vi "Force and Diameter Charts Notifier Debug.vi"(8 "error in (no error)":errorcluster, 9 "gui notifier":refnum<notifier>, 10 "error queue":refnum<queue>, 11 "ia test notifier":refnum<notifier>) -> (0 "error out":errorcluster)   [LabVIEW 2020]
uses:
  GUI/Main GUI Loop/Handler.ctl
  Inflation Test/Result Handling/Inflation Test Numeric Results.ctl
panel:
  out "diameter":cluster{dbl[], dbl[]}(graph)
  out "force vs setpoint":cluster{dbl[], dbl[]}[](graph)
  # "DIAMETER"
  # "FORCE VS. SETPOINT"
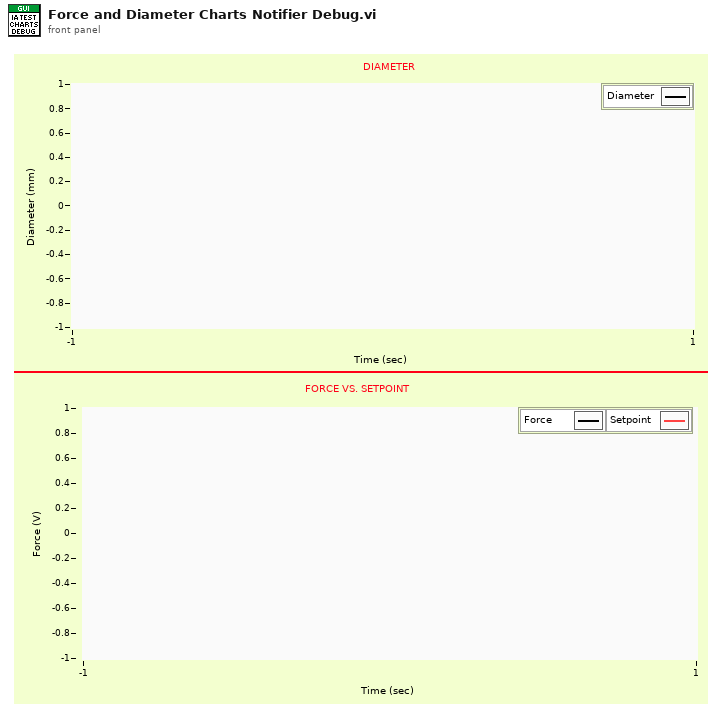
[diagram p1: front panel]
types:
  T1 = typedef "Inflation Test Numeric Results.ctl" = cluster{"diameter":dbl, "diam time":dbl, "force":dbl, "force time":dbl, "setpoint":dbl, "servo pw":dbl, "calibration log":dbl[][], "calibration results":dbl[][]}
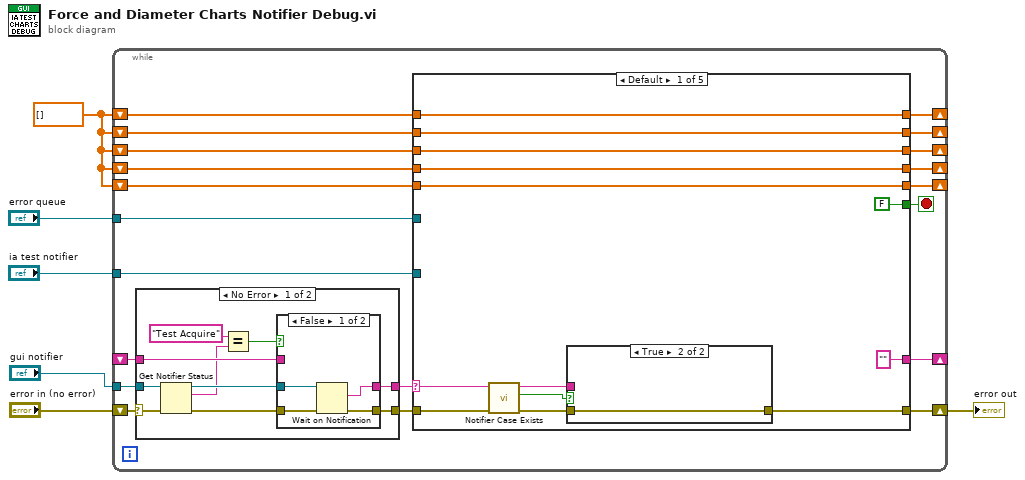
[diagram p0: block diagram]
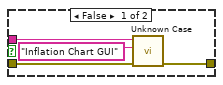
[diagram p2: hidden frame]
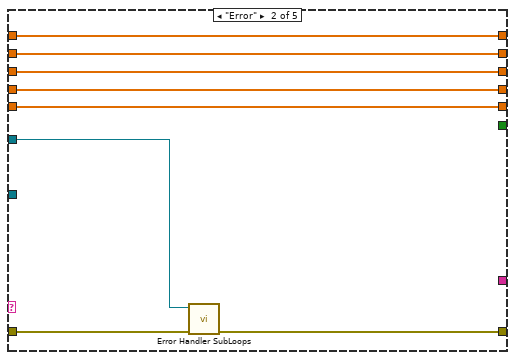
[diagram p3: hidden frame]
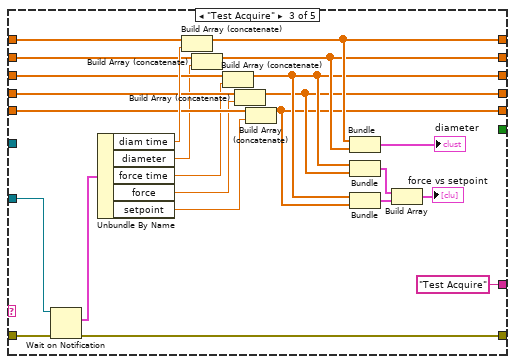
[diagram p4: hidden frame]
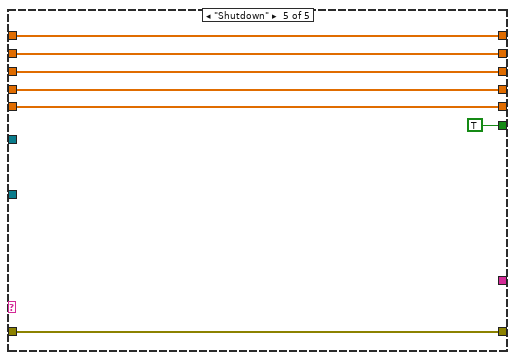
[diagram p6: hidden frame]
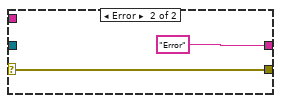
[diagram p8: hidden frame]
diagram:
  w1 = dbl[] [] ("appended array")
  n1 = while {
    tunnel: "ia test notifier" -> [w25]
    tunnel: "gui notifier" -> [w24]
    shift-right: [w21] -> w4
    shift-left: "error in (no error)" -> [w23]
    tunnel: "error queue" -> [w19]
    shift-right: [w13] -> _
    shift-left: w1 -> [w18]
    shift-right: [w12] -> _
    shift-left: w1 -> [w17]
    shift-right: [w11] -> _
    shift-left: w1 -> [w16]
    shift-right: [w10] -> _
    shift-left: w1 -> [w15]
    shift-right: [w9] -> _
    shift-left: w1 -> [w14]
    shift-right: [w8] -> _
    shift-left: _ -> [w7]
    stop <- w26 stop-if-true
    n2 = case shown="No Error" w23 {
      selector: w23 -> [w95 w107]
      tunnel: w24 -> [w93 _]
      tunnel: [w99 w107] -> w22
      tunnel: [w98 "Error" ("gui msg")] -> w20
      tunnel: w7 -> [w96 _]
      frame No Error {
        n3 = Get Notifier Status(notifier=w93, error in (no error)=w95) -> (notifier out=w92:refnum<notifier>, current notification=w91:string, error out=w94:errorcluster)  [unwired: 2 out]
        n4 = Equal?(x="Test Acquire" ("t"), y=w91) -> (x = y?=w90:bool)
        n5 = case shown="False" w90 {
          tunnel: w92 -> [w103 _]
          tunnel: [w102 w104] -> w99
          tunnel: w94 -> [w101 w104]
          tunnel: [w100 w105] -> w98
          tunnel: w96 -> [_ w105]
          frame False {
            n6 = Wait on Notification(notifier=w103, error in (no error)=w101) -> (notification=w100:string, error out=w102:errorcluster)  [unwired: 2 in, 2 out]
          }
          frame True {
          }
        }
      }
      frame Error {
      }
    }
    n7 = case shown="Default" w20 {
      selector: w20 -> [w29 _ _ _ _]
      tunnel: [FALSE _ _ _ TRUE] -> w26
      tunnel: w25 -> [_ _ w76 _ _]
      tunnel: w22 -> [w31 w46 w75 w77 w88]
      tunnel: [w38 w47 w74 w77 w88] -> w21
      tunnel: w19 -> [_ w45 _ _ _]
      tunnel: w18 -> [w33 w48 w72 w78 w87]
      tunnel: w17 -> [w34 w49 w70 w79 w86]
      tunnel: w16 -> [w35 w50 w69 w80 w85]
      tunnel: w15 -> [w36 w51 w68 w81 w84]
      tunnel: w14 -> [w37 w52 w67 w82 w83]
      tunnel: [w33 w48 w60 w78 w87] -> w13
      tunnel: [w34 w49 w59 w79 w86] -> w12
      tunnel: [w35 w50 w58 w80 w85] -> w11
      tunnel: [w36 w51 w57 w81 w84] -> w10
      tunnel: [w37 w52 w56 w82 w83] -> w9
      tunnel: ["" _ "Test Acquire" _ _] -> w8
      frame Default {
        n8 = call "Notifier Case Exists.vi"("error in (no error)"=w31, "case in"=w29) -> ("error out"=w30:errorcluster, "defined case?"=w27:bool, "case out"=w28:string)  [unwired: 7 in]
        n9 = case shown="True" w27 {
          tunnel: [w43 w44] -> w38
          tunnel: w30 -> [w41 w44]
          tunnel: w28 -> [w40 _]
          frame False {
            n10 = call "Unknown Case.vi"("error in (no error)"=w41, "source"="Inflation Chart GUI", "case"=w40) -> ("error out"=w43:errorcluster)  [unwired: 8 in]
          }
          frame True {
          }
        }
      }
      frame "Error" {
        n11 = call "Error Handler SubLoops.vi"("error in"=w46, "main gui queue"=w45) -> ("error out"=w47:errorcluster)  [unwired: 9 in]
      }
      frame "Test Acquire" {
        n12 = Wait on Notification(notifier=w76, error in (no error)=w75) -> (notification=w73:T1, error out=w74:errorcluster)  [unwired: 2 in, 2 out]
        n13 = Unbundle By Name(w73) -> ("diam time"=w71:dbl, "diameter"=w66:dbl, "force time"=w65:dbl, "force"=w64:dbl, "setpoint"=w63:dbl)
        n14 = Build Array (concatenate)(w72, w71) -> (w60:dbl[])
        n15 = Build Array (concatenate)(w70, w66) -> (w59:dbl[])
        n16 = Build Array (concatenate)(w69, w65) -> (w58:dbl[])
        n17 = Build Array (concatenate)(w68, w64) -> (w57:dbl[])
        n18 = Build Array (concatenate)(w67, w63) -> (w56:dbl[])
        n19 = Bundle(w60, w59) -> (→"diameter":cluster{dbl[], dbl[]})  [unwired: 1 in]
        n20 = Bundle(w58, w57) -> (w61:cluster{dbl[], dbl[]})  [unwired: 1 in]
        n21 = Bundle(w58, w56) -> (w62:cluster{dbl[], dbl[]})  [unwired: 1 in]
        n22 = Build Array(w61, w62) -> (→"force vs setpoint":cluster{dbl[], dbl[]}[])
      }
      frame "Stop Test GUI" {
      }
      frame "Shutdown" {
      }
    }
  }
  "error out" <- w4
